vi "Receiver.vi"() -> ()   [LabVIEW 2019]
uses:
  Data.ctl
  TypeDef/error.ctl
  Global - Pressure Data.vi
panel:
  out "ms":u32
  out "Numeric":i32
  out "length":i32
  out "open status":bool
  out "read error":errorcluster
  out "open error":errorcluster
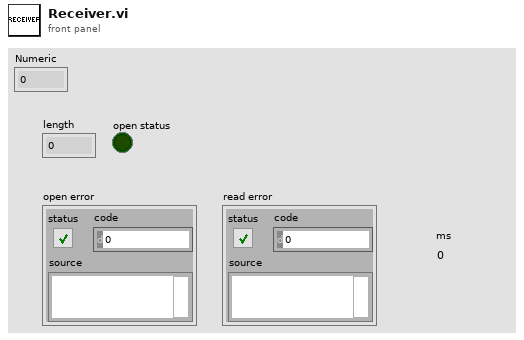
[diagram p1: front panel]
types:
  T1 = typedef "Data.ctl" = cluster{"P_DUT":dbl, "P_Chamber":dbl}
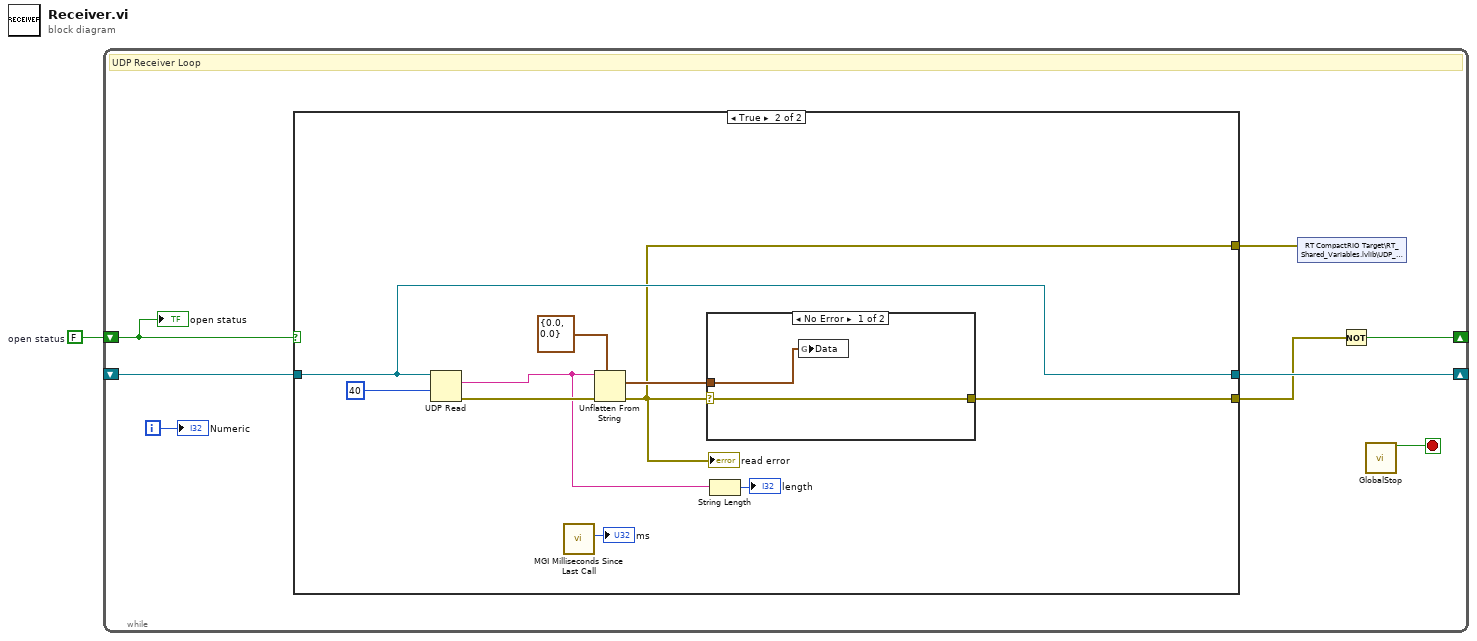
[diagram p0: block diagram]
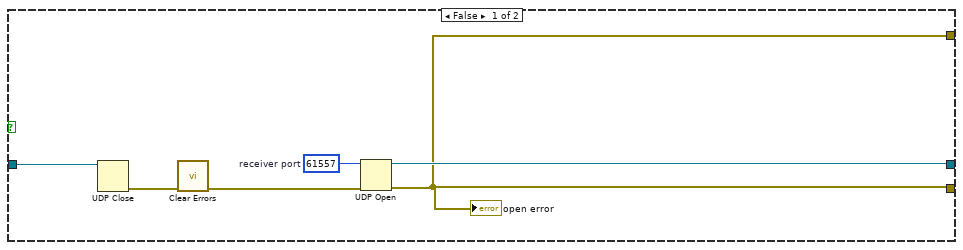
[diagram p2: hidden frame]
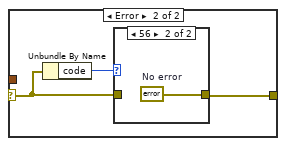
[diagram p4: hidden frame]
diagram:
  w1 = FALSE  # open status
  n1 = while {
    shift-right: [w8] -> _
    shift-left: _ -> [w9]
    shift-right: [w5] -> _
    shift-left: w1 -> [w7]
    i -> [w4]
    stop <- w3 stop-if-true
    # "UDP Receiver Loop"
    n2 = case shown="True" w7 {
      tunnel: w9 -> [w15 w18]
      tunnel: [w10 w19] -> w6
      tunnel: [w13 w18] -> w8
      tunnel: [w10 w16] -> w2
      frame False {
        w11 = u16 61557  # receiver port
        n3 = UDP Close(connection ID=w15) -> (error out=w14:errorcluster)  [unwired: 1 in, 1 out]
        n4 = call <vilib>:"Clear Errors.vi"("error in (no error)"=w14) -> ("error out"=w12:errorcluster)  [unwired: 5 in, 1 out]
        n5 = UDP Open(8:w12, 11:w11) -> (port=w13:refnum<k16>, 0:w10:errorcluster)  [unwired: 3 in, 1 out]
        "open error" <- w10
      }
      frame True {
        n6 = UDP Read(connection ID=w18, timeout ms (25000)=40) -> (data out=w21:string, error out=w24:errorcluster)  [unwired: 1 in, 4 out]
        n7 = call <userlib>:"MGI Milliseconds Since Last Call.vi"() -> ("ms"=→"ms":u32)  [unwired: 6 in, 1 out]
        n8 = Unflatten From String(type=T1 {"P_DUT"=0.0, "P_Chamber"=0.0} ("Data"), binary string=w21, error in (no error)=w24) -> (value=w22:T1, error out=w16:errorcluster)  [unwired: 2 in, 1 out]
        "read error" <- w16
        n9 = case shown="No Error" w16 {
          selector: w16 -> [w27 w35]
          tunnel: [w28 w34] -> w19
          tunnel: w22 -> [w26 _]
          frame No Error {
            n10 = global write "Global - Pressure Data.vi" "Data"(w26) -> ()
            n11 = disable-structure shown="Disabled" {
              disable-tunnel: _ -> [w33 _]
              disable-tunnel: [w32 _] -> w28
              disable-tunnel: [w31 _] -> _
              disable-tunnel: w27 -> [w30 _]
              frame Disabled {
                n12 = UDP Write(connection ID=w33, data in="OK", 8:w30) -> (error out=w32:errorcluster, 3:w31:refnum<k16>)  [unwired: 3 in]
              }
              frame Enabled {
              }
            }
          }
          frame Error {
            # "Sender did not send data. Ignore timeout error and keep waiting."
            n13 = Unbundle By Name(w35) -> ("code"=w36:i32)
            n14 = case shown="56" w36 {
              tunnel: w35 -> [w37 _]
              tunnel: [w37 w38] -> w34
              frame Default {
              }
              frame 56 {
                w38 = errorcluster {"status"=FALSE, "code"=0, "source"=""}  # No error
              }
            }
          }
        }
        n15 = String Length(string=w21) -> (length=→"length":i32)
      }
    }
    n16 = shared-variable "RT CompactRIO Target\\RT_Shared_Variables.lvlib\\UDP_ERROR"(w2) -> ()  [unwired: 1 in, 1 out]
    n17 = Not(x=w6) -> (.not. x?=w5:bool)
    n18 = call "GlobalStop.vi"() -> ("Stop"=w3:bool)  [unwired: 15 in]
    "open status" <- w7
    "Numeric" <- w4
  }
